vi "Create_Trajectory_Check_Diff_Drive_Max_Speed.vi"(6 "Use Diff Drive\nKinematic\nConstraint":bool, 9 "Max Speed M/S":dbl, 10 "DIFF_DRIVE_KINEMATICS":T1 {"TrackWidth_Meters" format="%20.4f"}, 11 "States":T2[](array[typedef]) {"POSE"."ROTATION"."SIN" format="%13.4f"; "POSE"."ROTATION"."COS" format="%13.4f"; "POSE"."ROTATION"."VALUE" format="%13.4f"; "POSE"."TRANSLATION"."Y" format="%14.3f"; "POSE"."TRANSLATION"."X" format="%14.3f"}) -> (2 "Inches/Second":dbl, 3 "Max Speed Exceeded":bool)   [LabVIEW 2019]
uses:
  <vilib>/Rock Robotics/WPI/ThirdParty/JAS_Junk/TrajLib/Trajectory_Library.lvlib
  <vilib>/Rock Robotics/WPI/ThirdParty/JAS_Junk/TrajLib/TRANSLATION2D.ctl
  <vilib>/Rock Robotics/WPI/ThirdParty/JAS_Junk/TrajLib/ROTATION2D.ctl
  <vilib>/Rock Robotics/WPI/ThirdParty/JAS_Junk/TrajLib/POSE2D.ctl
  <vilib>/Rock Robotics/WPI/ThirdParty/JAS_Junk/TrajLib/TRAJ_STATE.ctl
  <vilib>/Rock Robotics/WPI/ThirdParty/JAS_Junk/TrajLib/DIFF_DRIVE_KINEMATICS.ctl
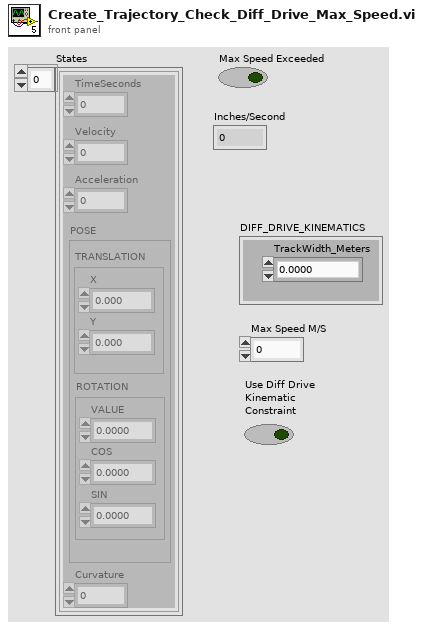
[diagram p1: front panel]
types:
  T1 = typedef "Trajectory_Library.lvlib/DIFF_DRIVE_KINEMATICS.ctl" = cluster{"TrackWidth_Meters":dbl}
  T2 = typedef "Trajectory_Library.lvlib/TRAJ_STATE.ctl" = cluster{"TimeSeconds":dbl, "Velocity":dbl, "Acceleration":dbl, "POSE":T3, "Curvature":dbl}
  T3 = typedef "Trajectory_Library.lvlib/POSE2D.ctl" = cluster{"TRANSLATION":T4, "ROTATION":T5}
  T4 = typedef "Trajectory_Library.lvlib/TRANSLATION2D.ctl" = cluster{"X":dbl, "Y":dbl}
  T5 = typedef "Trajectory_Library.lvlib/ROTATION2D.ctl" = cluster{"VALUE":dbl, "COS":dbl, "SIN":dbl}
  T6 = typedef "Trajectory_Library.lvlib/CHASSIS_SPEEDS.ctl" = cluster{"vX":dbl, "vY":dbl, "vOmega":dbl}
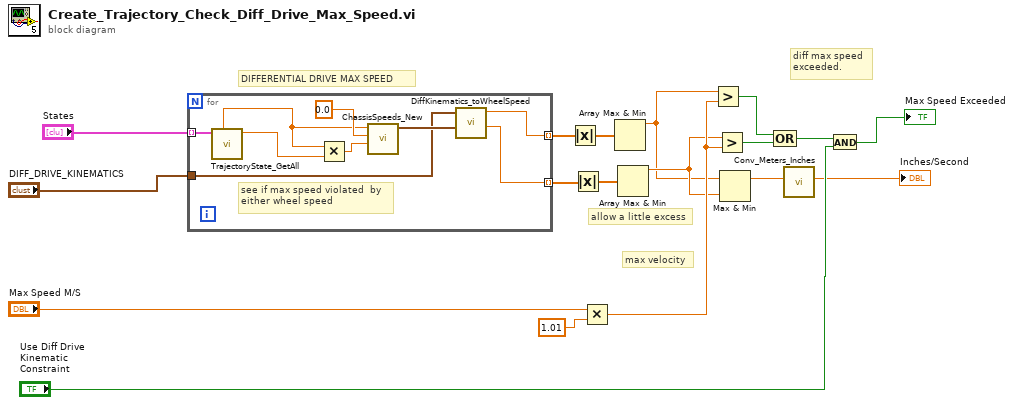
[diagram p0: block diagram]
diagram:
  # "diff max speed\nexceeded."
  # "max velocity"
  # "allow a little excess"
  # "DIFFERENTIAL DRIVE MAX SPEED"
  n1 = for {
    tunnel: [w23] -> w2 mode=indexing
    tunnel: [w22] -> w4 mode=indexing
    tunnel: "States" -> [w21] mode=indexing
    tunnel: "DIFF_DRIVE_KINEMATICS" -> [w24]
    # "see if max speed violated  by\neither wheel speed"
    n2 = call <vilib>:"TrajectoryState_GetAll.vi"("TRAJ_STATE"=w21) -> ("Curvature"=w19:dbl, "Velocity"=w20:dbl)  [unwired: 4 in, 5 out]
    n3 = Multiply(x=w20, y=w19) -> (x*y=w26:dbl)
    n4 = call <vilib>:"ChassisSpeeds_New.vi"("vAngular"=w26, "vY"=0.0, "vX"=w20) -> ("CHASSIS"=w25:T6)  [unwired: 8 in]
    n5 = call <vilib>:"DiffKinematics_toWheelSpeed.vi"("CHASSIS Speed"=w25, "DIFF_DRIVE_KINEMATICS"=w24) -> ("RightVelocity"=w22:dbl, "LeftVelocity"=w23:dbl)  [unwired: 8 in]
  }
  n6 = Absolute Value(x=w2) -> (abs(x)=w3:dbl[])
  n7 = Absolute Value(x=w4) -> (abs(x)=w5:dbl[])
  n8 = Multiply(x="Max Speed M/S", y=1.01) -> (x*y=w13:dbl)
  n9 = Array Max & Min(array=w3) -> (max value=w7:dbl)  [unwired: 3 out]
  n10 = Array Max & Min(array=w5) -> (max value=w8:dbl)  [unwired: 3 out]
  n11 = Greater?(x=w7, y=w13) -> (0:w1:bool)
  n12 = Greater?(x=w8, y=w13) -> (0:w6:bool)
  n13 = Max & Min(x=w7, y=w8) -> (max(x,y)=w10:dbl)  [unwired: 1 out]
  n14 = Compound Arithmetic op=OR(w1, w6) -> (w15:bool)
  n15 = call <vilib>:"Conv_Meters_Inches.vi"("Meters"=w10) -> ("Inches"=→"Inches/Second":dbl)  [unwired: 10 in]
  n16 = And(x=w15, y="Use Diff Drive\nKinematic\nConstraint") -> (x .and. y?=→"Max Speed Exceeded":bool)
